vi "Decode SSL Wrapper Package.vi"(5 "Version":string(combo)="Auto", 8 "error in (no error)":errorcluster, 11 "unsigned byte array":u8[](array[numeric])) -> (0 "error out":errorcluster, 1 "Geometry Camera Calibration":T2, 2 "Field Size":T1, 3 "Detection Frame":T3 {"robots_blue"."height" format="%+4.3f"; "robots_blue"."pixel_y" format="%+4.3f"; "robots_blue"."pixel_x" format="%+4.3f"; "robots_blue"."orientation" format="%+4.3f"; "robots_blue"."y" format="%+4.3f"; "robots_blue"."confidence" format="%4.3f"; "robots_blue"."x" format="%+4.3f"; "robots_yellow"."height" format="%+4.3f"; "robots_yellow"."pixel_y" format="%+4.3f"; "robots_yellow"."pixel_x" format="%+4.3f"; "robots_yellow"."orientation" format="%+4.3f"; "robots_yellow"."y" format="%+4.3f"; "robots_yellow"."confidence" format="%4.3f"; "robots_yellow"."x" format="%+4.3f"})   [LabVIEW 2017]
uses:
  SSL Detection Robot.ctl
  SSL Detection Ball.ctl
  SSL Detection Frame.ctl
  SSL Geometry Camera Calibration.ctl
  <vilib>/Analysis/Matrix/Datatypes/RealMatrix.ctl
  <vilib>/Analysis/Matrix/NI_Matrix.lvlib
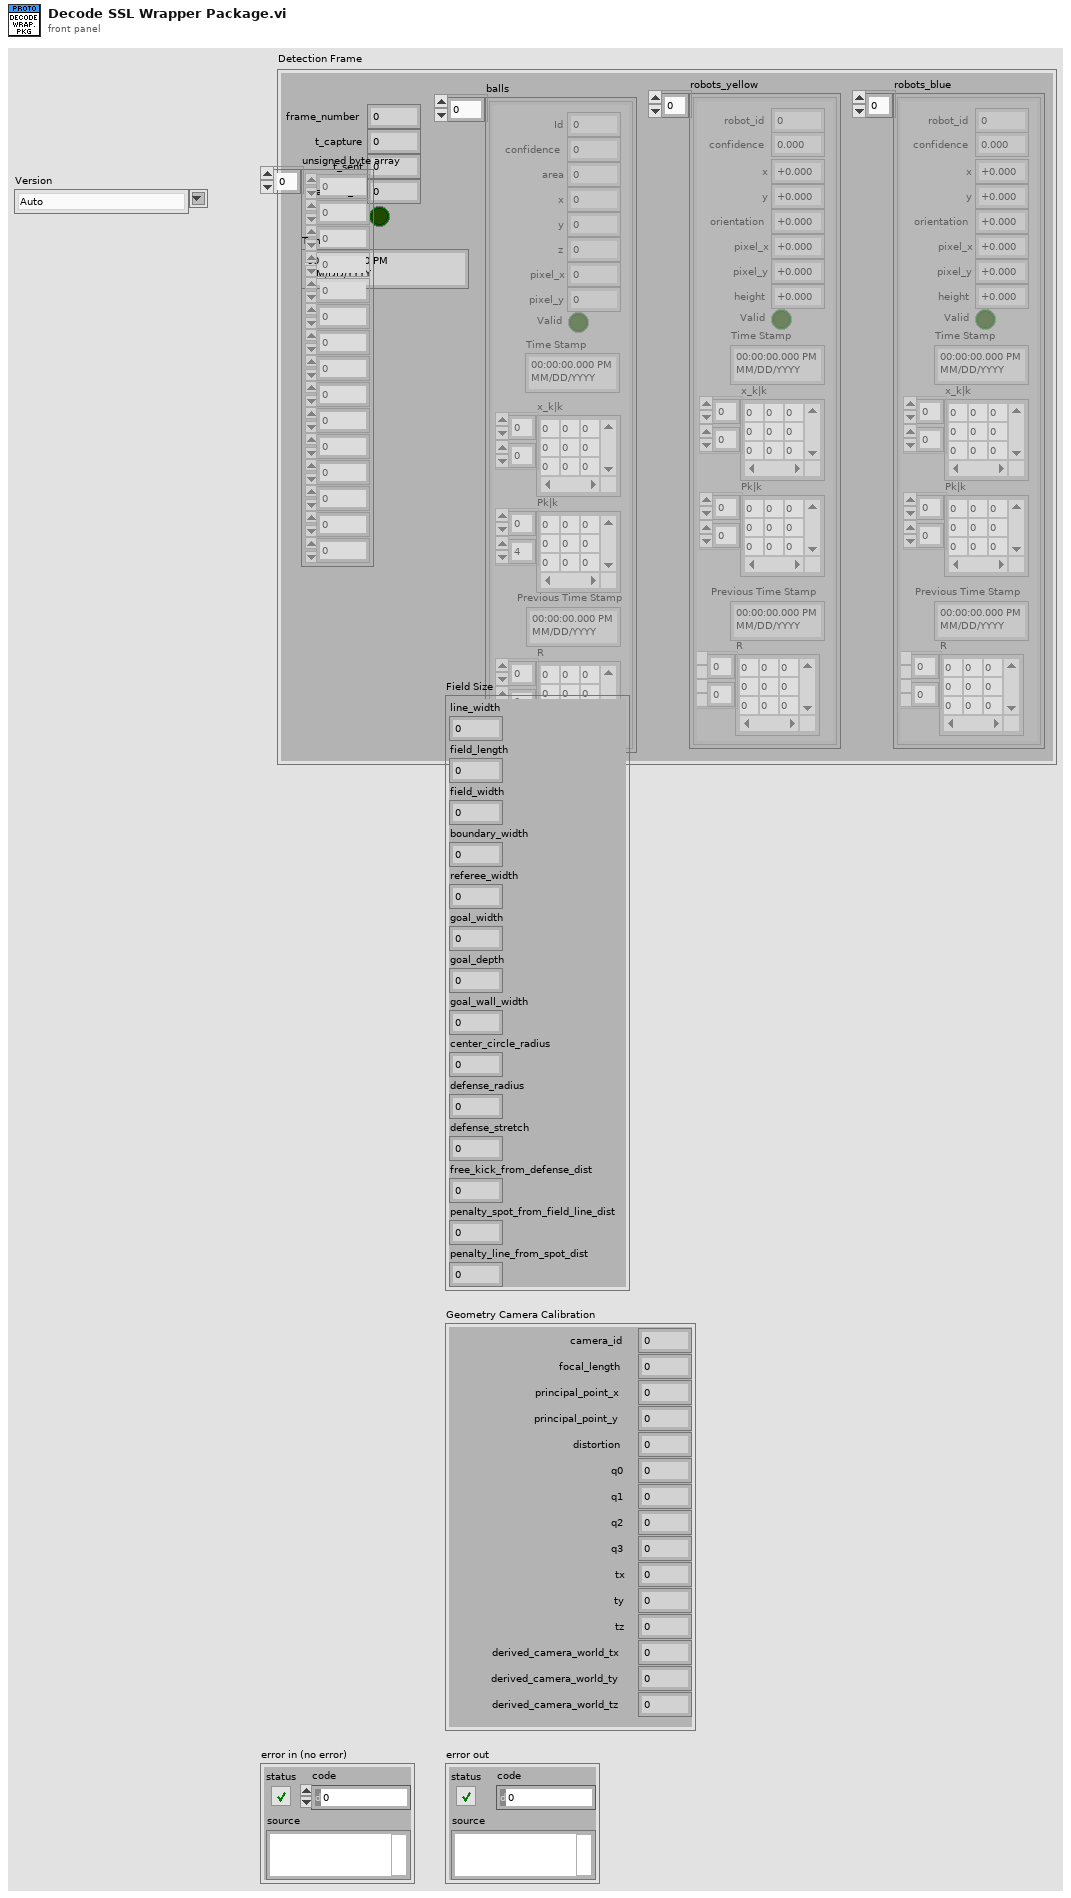
[diagram p1: front panel]
types:
  T1 = cluster{"line_width":u32, "field_length":u32, "field_width":u32, "boundary_width":u32, "referee_width":u32, "goal_width":u32, "goal_depth":u32, "goal_wall_width":u32, "center_circle_radius":u32, "defense_radius":u32, "defense_stretch":u32, "free_kick_from_defense_dist":u32, "penalty_spot_from_field_line_dist":u32, "penalty_line_from_spot_dist":u32}
  T2 = typedef "SSL Geometry Camera Calibration.ctl" = cluster{"camera_id":u32, "focal_length":sgl, "principal_point_x":sgl, "principal_point_y":sgl, "distortion":sgl, "q0":sgl, "q1":sgl, "q2":sgl, "q3":sgl, "tx":sgl, "ty":sgl, "tz":sgl, "derived_camera_world_tx":sgl, "derived_camera_world_ty":sgl, "derived_camera_world_tz":sgl}
  T3 = typedef "SSL Detection Frame.ctl" = cluster{"frame_number":u32, "t_capture":dbl, "t_sent":dbl, "camera_id":u32, "robots_yellow":T4[], "robots_blue":T4[], "balls":T6[], "Valid":bool, "Time Stamp":timestamp}
  T4 = typedef "SSL Detection Robot.ctl" = cluster{"x":sgl, "robot_id":u32, "confidence":sgl, "y":sgl, "orientation":sgl, "pixel_x":sgl, "pixel_y":sgl, "height":sgl, "Valid":bool, "Time Stamp":timestamp, "x_k|k":T5, "Pk|k":T5, "Previous Time Stamp":timestamp, "R":T5}
  T5 = typedef "NI_Matrix.lvlib/RealMatrix.ctl" = dbl[][]
  T6 = typedef "SSL Detection Ball.ctl" = cluster{"x":sgl, "area":u32, "confidence":sgl, "y":sgl, "z":sgl, "pixel_x":sgl, "pixel_y":sgl, "Valid":bool, "Time Stamp":timestamp, "x_k|k":T5, "Pk|k":T5, "Id":u32, "Previous Time Stamp":timestamp, "R":T5}
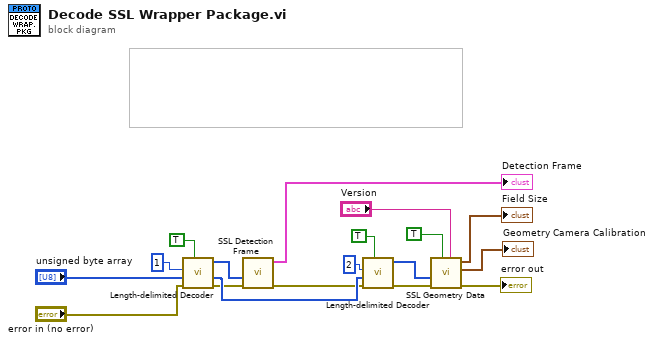
[diagram p0: block diagram]
diagram:
  n1 = call "Length-delimited Decoder.vi"("Optional"=TRUE, "error in (no error)"="error in (no error)", "Array"="unsigned byte array", "Key"=1) -> ("error out"=w4:errorcluster, "array w/ subset deleted"=w11:u8[], "Length-delimited"=w10:u8[])  [unwired: 4 in, 1 out]
  n2 = call "SSL Detection Frame.vi"("error in"=w4, "Array"=w10) -> ("error out"=w5:errorcluster, "Detection Frame"=→"Detection Frame":T3)  [unwired: 8 in]
  n3 = call "Length-delimited Decoder.vi"("Optional"=TRUE, "error in (no error)"=w5, "Array"=w11, "Key"=2) -> ("error out"=w8:errorcluster, "Length-delimited"=w15:u8[])  [unwired: 4 in, 2 out]
  n4 = call "SSL Geometry Data.vi"("Version"="Version", "Optional"=TRUE, "error in"=w8, "Array"=w15) -> ("error out"=→"error out":errorcluster, "Geometry Camera Calibration"=→"Geometry Camera Calibration":T2, "Field Size"=→"Field Size":T1)  [unwired: 5 in]
